vi "sample obtain bucket and list objects.vi"() -> ()   [LabVIEW 2015]
uses:
  Object Content.ctl
  Storage Class.ctl
  Owner.ctl
  Core/HTTP Request/AWS Credentials.ctl
  Bucket/Bucket.lvclass
  Core/HTTP Request/HTTP Request.lvclass
  NI_AWS_S3.lvlib
panel:
  out "Objects":T1[](array[typedef])
  out "error out":errorcluster
  in  "Bucket name":string="bpreis-test-96"
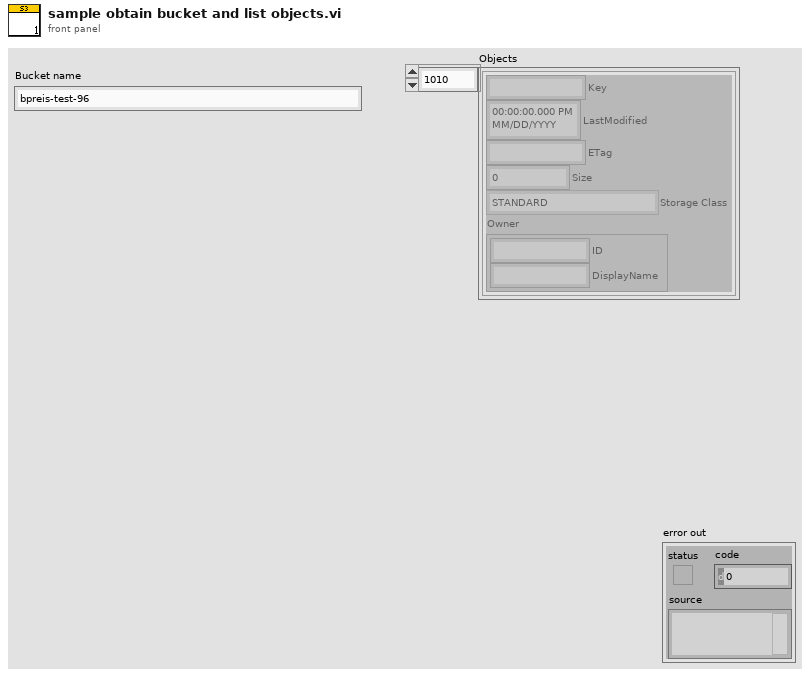
[diagram p1: front panel]
types:
  T1 = typedef "NI_AWS_S3.lvlib/Object Content.ctl" = cluster{"Key":string, "LastModified":timestamp, "ETag":string, "Size":u64, "Storage Class":T2, "Owner":T3}
  T2 = typedef "NI_AWS_S3.lvlib/Storage Class.ctl" = enum16{"STANDARD", "REDUCED_REDUNDANCY"}
  T3 = typedef "NI_AWS_S3.lvlib/Owner.ctl" = cluster{"ID":string, "DisplayName":string}
  T4 = typedef "NI_AWS_Core.lvlib/HTTP Request.lvclass/AWS Credentials.ctl" = cluster{"Access Key":string, "Secret Key":string}
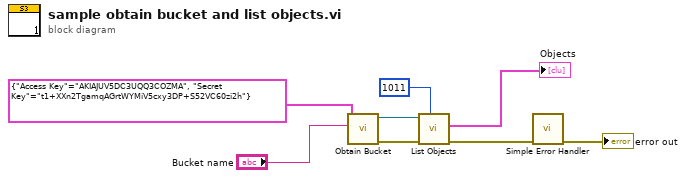
[diagram p0: block diagram]
diagram:
  n1 = call "Obtain Bucket.vi"("Bucket name"="Bucket name", "AWS Credentials"=T4 {"Access Key"="AKIAJUV5DC3UQQ3COZMA", "Secret Key"="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"}) -> ("error out"=w5:errorcluster, "Bucket"=w6:refnum<class "Bucket.lvclass">)  [unwired: 8 in]
  n2 = call "List Objects.vi"("Max keys"=u32 1011, "error in (no error)"=w5, "Bucket in"=w6) -> ("error out"=w3:errorcluster, "Objects"=→"Objects":T1[])  [unwired: 5 in, 2 out]
  n3 = call <vilib>:"Simple Error Handler.vi"("error in (no error)"=w3) -> ("error out"=→"error out":errorcluster)  [unwired: 4 in, 4 out]
